vi "Fixed Channel Module Script.vi"   [LabVIEW 2013]
uses:
  fixed module parent/script/FromClusterToTagBusScript.vi
  fixed module parent/script/data interface script.lvlib
types:
  T1 = enum32{"Invalid", "Standard", "Closed", "Hidden", "Minimized", "Maximized"}
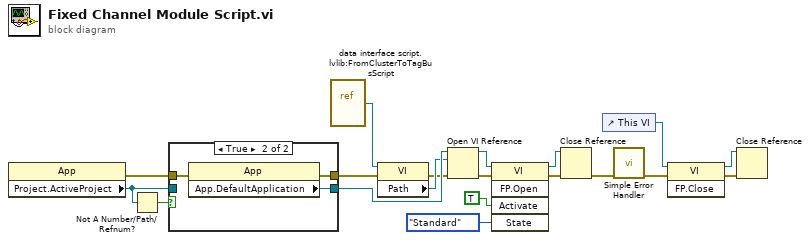
[diagram p0: block diagram]
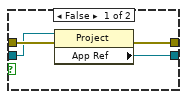
[diagram p2: hidden frame]
diagram:
  n1 = property class="App"() -> (error out=w18:errorcluster, "Project.ActiveProject"=w7:refnum<vi>)  [unwired: 2 in, 1 out]
  n2 = Not A Number/Path/Refnum?(number/path/refnum=w7) -> (NaN/Path/Refnum?=w6:bool)
  n3 = case shown="True" w6 {
    tunnel: w18 -> [w23 w26]
    tunnel: [w22 w24] -> w17
    tunnel: [w21 w25] -> w14
    tunnel: w7 -> [w20 _]
    frame False {
      n4 = property class="Project"(reference=w20, error in=w23) -> (error out=w21:errorcluster, "App Ref"=w22:refnum<vi>)  [unwired: 1 out]
    }
    frame True {
      n5 = property class="App"(error in=w26) -> (error out=w25:errorcluster, "App.DefaultApplication"=w24:refnum<vi>)  [unwired: 1 in, 1 out]
    }
  }
  n6 = vi-ref "data interface script.lvlib:FromClusterToTagBusScript.vi"() -> (w19:refnum<vi>)
  n7 = property class="VI"(reference=w19, error in=w14) -> (error out=w15:errorcluster, "Path"=w16:path)  [unwired: 1 out]
  n8 = Open VI Reference(application reference (local)=w17, vi path=w16, error in (no error)=w15) -> (vi reference=w12:refnum<vi>, error out=w13:errorcluster)  [unwired: 3 in]
  n9 = invoke class="VI" method="FP.Open"(reference=w12, error in=w13, "Activate"=TRUE ("Activate?"), "State"=T1."Standard") -> (reference out=w10:refnum<vi>, error out=w11:errorcluster)  [unwired: 1 in, 3 out]
  n10 = Close Reference(reference=w10, error in (no error)=w11) -> (error out=w5:errorcluster)
  n11 = control-ref of="This VI"() -> (w3:refnum<vi>)
  n12 = call <vilib>:"Simple Error Handler.vi"("error in (no error)"=w5) -> ("error out"=w4:errorcluster)  [unwired: 4 in, 4 out]
  n13 = invoke class="VI" method="FP.Close"(reference=w3, error in=w4) -> (reference out=w1:refnum<vi>, error out=w2:errorcluster)  [unwired: 1 in, 1 out]
  n14 = Close Reference(reference=w1, error in (no error)=w2) -> ()  [unwired: 1 out]
